vi "driveable_paths_behavior.vi"() -> ()   [LabVIEW 2009]
uses:
  <vilib>/Platform/TimedLoop/XDataNode/XDataNode.xnode
  <vilib>/Platform/TimedLoop/XDataNode/loadlvalarms.vi
  <vilib>/Platform/TimedLoop/XDataNode/timing_clust.ctl
  <vilib>/Platform/TimedLoop/XDataNode/nitl_modes.ctl
  <vilib>/Platform/TimedLoop/XDataNode/wakeup.ctl
  <vilib>/Platform/TimedLoop/XDataNode/XDNodeRunTimeDep.lvlib
panel:
  in  "x LIDAR position":i16
  in  "y LIDAR position":i16
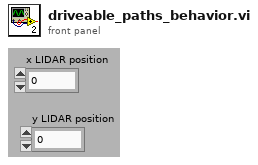
[diagram p1: front panel]
types:
  T1 = typedef "XDNodeRunTimeDep.lvlib/timing_clust.ctl" = cluster{"Expected End [f-1]":u64, "Actual End [f-1]":u64, "Finished Late? [f-1]":bool, "Expected End [i-1]":u64, "Actual End [i-1]":u64, "Finished Late? [i-1]":bool, "Expected Start [i]":u64, "Actual Start [i]":u64, "Expected Start [f]":u64, "Actual Start [f]":u64, "Source Name":string, "Structure Name":string, "Period":i64, "Deadline":i64, "Offset":i64, "Start":i64, "Priority":i32, "Timeout":i32, "Mode":T2, "Wakeup Reason":T3, "Error":errorcluster, "Source Type":string, "Secondary Source Type":string, "Global End Time":u64, "Global Start Time":u64, "Frame Duration":u64, "Iteration Duration":u64, "Assigned CPU":i32, "I/O Scan Engine Mode":u32}
  T2 = typedef "XDNodeRunTimeDep.lvlib/nitl_modes.ctl" = enum32{"No Change", "Process missed periods, maintain original phase", "Discard missed periods, maintain original phase", "Process missed periods, ignore original phase", "Discard missed periods, ignore original phase"}
  T3 = typedef "XDNodeRunTimeDep.lvlib/wakeup.ctl" = enum32{"Normal", "Aborted", "Asynchronous wakeup", "Timing source error", "Timed loop error", "Timeout"}
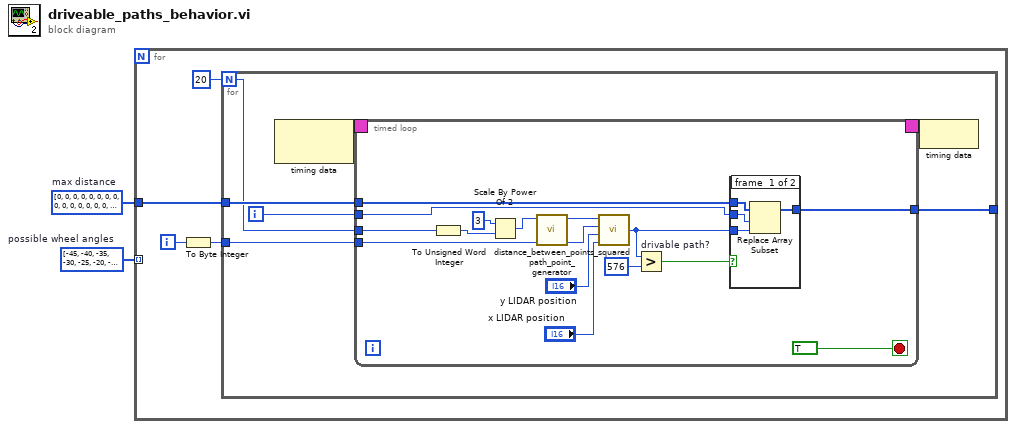
[diagram p0: block diagram]
diagram:
  w1 = i8[] [-45, -40, -35, -30, -25, -20, -15, -10, -5, 0, 5, 10, 15, 20, 25, 30, 35, 40, 45]  # possible wheel angles
  w2 = i16[] [0, 0, 0, 0, 0, 0, 0, 0, 0, 0, 0, 0, 0, 0, 0, 0, 0, 0, 0]  # max distance
  n1 = for {
    tunnel: w2 -> [w6]
    tunnel: w1 -> [_] mode=indexing
    i -> [w4]
    n2 = To Byte Integer(number=w4) -> (8bit integer=w3:i8)
    n3 = for {
      N: 20 -> [w10]
      tunnel: w6 -> [w13]
      tunnel: [w11] -> _
      tunnel: w3 -> [w9]
      i -> [w12]
      n4 = node-c288() -> (w8:T1)  [unwired: 1 in]
      n5 = timed-loop {
        timing: w8 -> [_]
        timing-out: [_] -> w7
        tunnel: w13 -> [w29]
        tunnel: w12 -> [w28]
        tunnel: [w27] -> w11
        tunnel: w10 -> [w26]
        tunnel: w9 -> [w20]
        stop <- TRUE stop-if-true
        n6 = To Unsigned Word Integer(number=w26) -> (unsigned 16bit integer=w24:u16)
        n7 = Scale By Power Of 2(n=u16 3, x=w24) -> (x*2^n=w21:u16)
        n8 = call "path_point_generator.vi"("wheel angle"=w20, "distance"=w21) -> ("y position"=w22:i16, "x position"=w23:i16)  [unwired: 8 in]
        n9 = call "distance_between_points_squared.vi"("x LIDAR position"="x LIDAR position", "y LIDAR position"="y LIDAR position", "x position"=w22, "y position"=w23) -> ("distance squared"=w15:i16)  [unwired: 2 in]
        n10 = Greater? "drivable path?"(x=w15, y=i16 576) -> (0:w16:bool)
        n11 = case shown="True" w16 {
          tunnel: w29 -> [w33 w34]
          tunnel: w28 -> [w32 _]
          tunnel: w15 -> [w31 _]
          tunnel: [w30 w34] -> w27
          frame #0 {
            n12 = Replace Array Subset(array=w33, new element=w31, index=w32) -> (w30:i16[])
          }
          frame #1 {
          }
        }
      }
      n13 = node-c288(w7) -> ()
    }
  }
